vi "CFTS-Connections Dialog.vi"(2 "Parent VI":refnum<vi>) -> ()   [LabVIEW 2020]
doc: "Use this template to create a dialog box with event handling."
uses:
  epl-vi-lib/Utility VIs/Controls/KBackground Gradient/KBackground Gradient.xctl
  epl-vi-lib/Utility VIs/Controls/KTable/KTable.xctl
  CFTS-Options.ctl
  epl-vi-lib/Connection VIs/Typedefs/CM-Endpoint.ctl
  76337d95-708c-4186-8447-1f4ad4f75f43.vi
  epl-vi-lib/Utility VIs/File IO VIs/Read Write Anything/Read Anything.vi
panel:
  in  "TermConfig":bool
  in  "AO":u16(xcontrol)
  in  "AI":u16(xcontrol)
  in  "background":dbl(xcontrol)
  in  "Cancel":bool
  in  "OK":bool
  # "Connections"
  # "Outputs"
  # "Inputs"
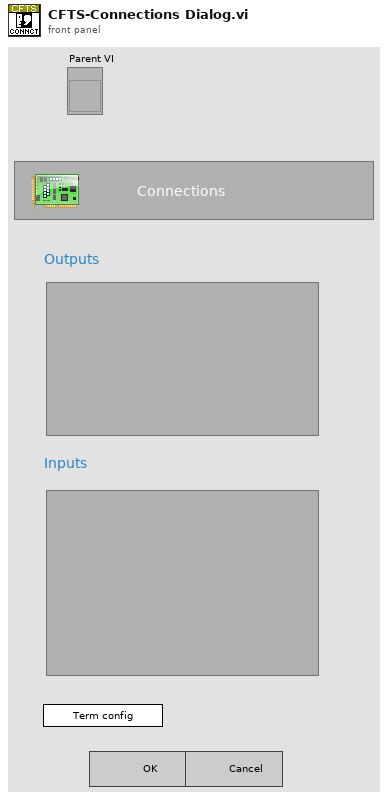
[diagram p1: front panel]
types:
  T1 = typedef "CFTS-Options.ctl" = cluster{"Rig ID":string, "Acoustic System IDs":cluster{"Right":string, "Left":string}, "Extension":string, "Advanced users":string[], "All advanced":bool, "Run vitals":bool, "hash":string, "Allow nonEPL":bool, "NonEPL":string[], "Data root":path}
  T2 = typedef "CM-Endpoint.ctl" = cluster{"Name":string, "Device":string}
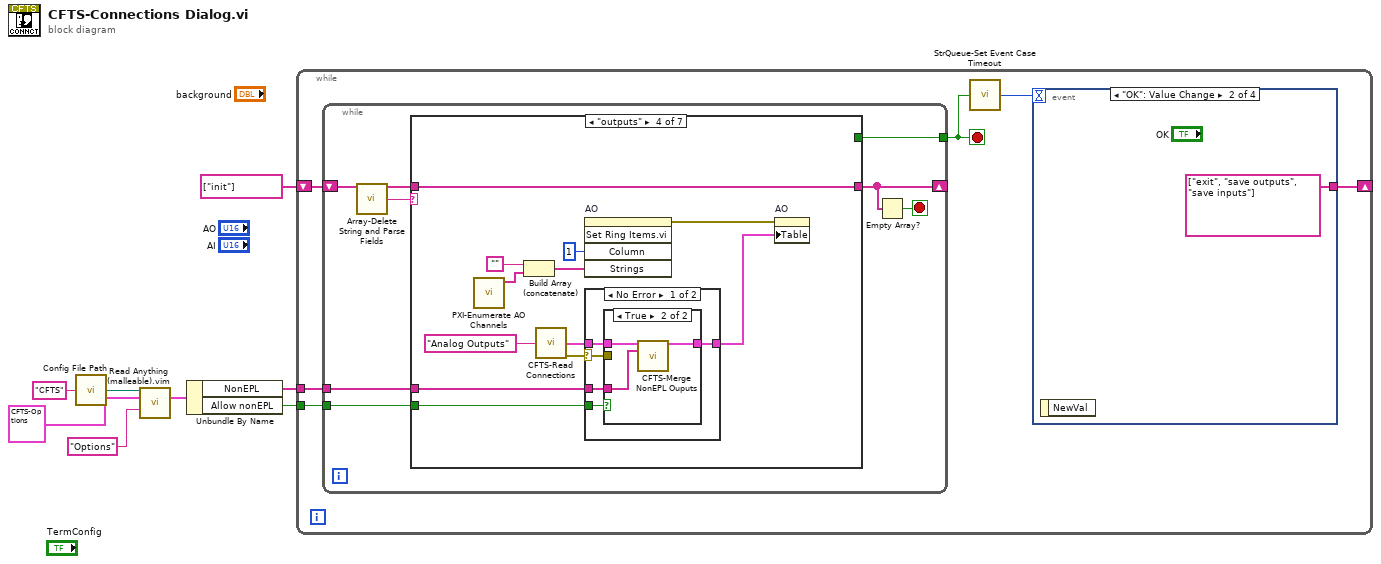
[diagram p0: block diagram]
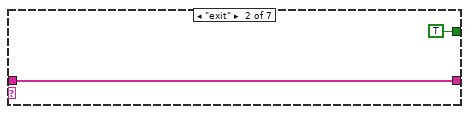
[diagram p3: hidden frame]
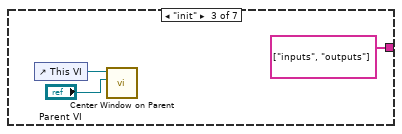
[diagram p4: hidden frame]
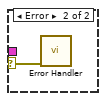
[diagram p6: hidden frame]
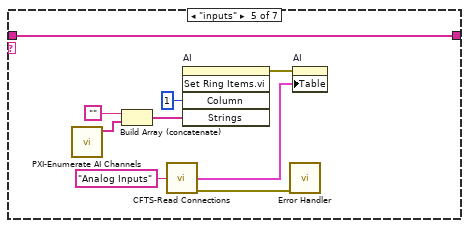
[diagram p7: hidden frame]
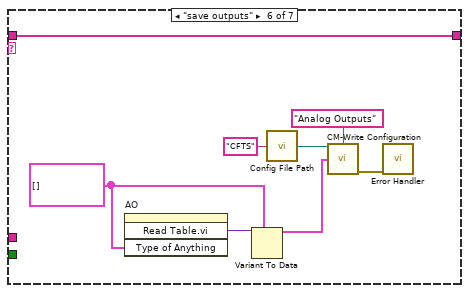
[diagram p8: hidden frame]
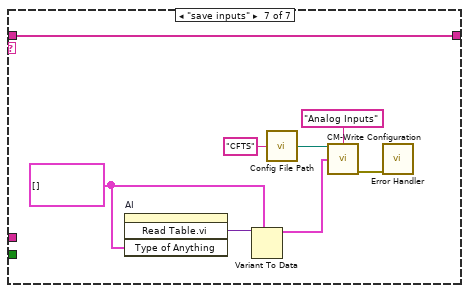
[diagram p9: hidden frame]
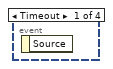
[diagram p10: hidden frame]
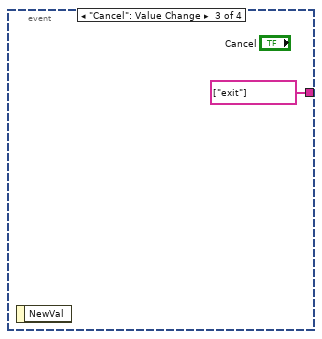
[diagram p11: hidden frame]
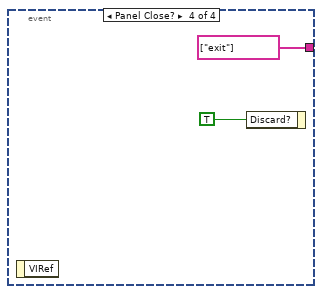
[diagram p12: hidden frame]
diagram:
  n1 = call "Config File Path.vi"("AppName"="CFTS") -> ("Default config file name"=w6:path)
  n2 = call "Read Anything (malleable).vim"("Config file path"=w6, "Options in"=T1 {"Rig ID"="", "Acoustic System IDs"={"Right"="", "Left"=""}, "Extension"="", "Advanced users"=[], "All advanced"=FALSE, "Run vitals"=FALSE, "hash"="", "Allow nonEPL"=FALSE, "NonEPL"=[], "Data root"=path ""} ("Options"), "Section"="Options") -> ("Options out"=w3:T1)  [unwired: 9 in, 3 out]
  n3 = Unbundle By Name(w3) -> ("NonEPL"=w2:string[], "Allow nonEPL"=w1:bool)
  n4 = while {
    shift-right: [w11] -> _
    shift-left: string[] ["init"] -> [w12]
    tunnel: w2 -> [w10]
    tunnel: w1 -> [w9]
    stop <- w14 stop-if-true
    n5 = while {
      shift-right: [w22] -> _
      shift-left: w12 -> [w19]
      tunnel: [w20] -> w14
      tunnel: w10 -> [w16]
      tunnel: w9 -> [w15]
      stop <- w21 stop-if-true
      n6 = call "Array-Delete String and Parse Fields.vi"("Array in"=w19) -> ("Array out"=w18:string[], "Field 1"=w17:string)  [unwired: 10 in, 3 out]
      n7 = case shown="\"outputs\"" w17 {
        tunnel: w18 -> [w23 w25 _ w40 w59 w67 w75]
        tunnel: [w23 w25 string[] ["inputs", "outputs"] ("Array out") w40 w59 w67 w75] -> w22
        tunnel: [_ TRUE _ _ _ _ _] -> w20
        tunnel: w16 -> [_ _ _ w29 _ _ _]
        tunnel: w15 -> [_ _ _ w32 _ _ _]
        frame "", Default {
        }
        frame "exit" {
        }
        frame "init" {
          n8 = control-ref of="This VI"() -> (w27:refnum<vi>)
          n9 = call "Center Window on Parent.vi"("Parent VI"="Parent VI", "VI in"=w27) -> ()  [unwired: 8 in, 2 out]
        }
        frame "outputs" {
          n10 = call "PXI-Enumerate AO Channels.vi"() -> ("AO.PhysicalChans"=w37:tag[])  [unwired: 10 in, 1 out]
          n11 = Build Array (concatenate)("", w37) -> (w35:string[])
          n12 = call "CFTS-Read Connections.vi"("Which"="Analog Outputs") -> ("endpoints"=w31:T2[], "error out"=w33:errorcluster)  [unwired: 13 in]
          n13 = invoke on="AO" class="KTable (strict)" method="Set Ring Items.vi"("Column"=1, "Strings"=w35) -> (error out=w39:errorcluster)  [unwired: 3 in, 4 out]
          n14 = case shown="No Error" w33 {
            selector: w33 -> [w45 w50]
            tunnel: w32 -> [w44 _]
            tunnel: w31 -> [w43 _]
            tunnel: [w42 _] -> w30
            tunnel: w29 -> [w41 _]
            frame No Error {
              n15 = case shown="True" w44 {
                tunnel: w45 -> [_ _]
                tunnel: w43 -> [w46 w47]
                tunnel: [w46 w48] -> w42
                tunnel: w41 -> [_ w49]
                frame False {
                }
                frame True {
                  n16 = call "CFTS-Merge NonEPL Ouputs.vi"("endpoints in"=w47, "NonEPL"=w49) -> ("endpoints out"=w48:T2[])  [unwired: 13 in]
                }
              }
            }
            frame Error {
              n17 = call "Error Handler.vi"("error in (no error)"=w50) -> ()  [unwired: 12 in, 3 out]
            }
          }
          n18 = property on="AO" class="KTable (strict)"(error in=w39, "Table"=w30) -> ()  [unwired: 1 in, 2 out]
        }
        frame "inputs" {
          n19 = call "PXI-Enumerate AI Channels.vi"() -> ("AI.PhysicalChans"=w56:tag[])  [unwired: 11 in]
          n20 = Build Array (concatenate)("", w56) -> (w54:string[])
          n21 = call "CFTS-Read Connections.vi"("Which"="Analog Inputs") -> ("endpoints"=w52:T2[], "error out"=w53:errorcluster)  [unwired: 13 in]
          n22 = invoke on="AI" class="KTable (strict)" method="Set Ring Items.vi"("Column"=1, "Strings"=w54) -> (error out=w58:errorcluster)  [unwired: 3 in, 4 out]
          n23 = call "Error Handler.vi"("error in (no error)"=w53) -> ()  [unwired: 12 in, 3 out]
          n24 = property on="AI" class="KTable (strict)"(error in=w58, "Table"=w52) -> ()  [unwired: 1 in, 2 out]
        }
        frame "save outputs" {
          w64 = T2[] [] ("Array")
          n25 = invoke on="AO" class="KTable (strict)" method="Read Table.vi"("Type of Anything"=w64) -> ("Read Table.vi"=w65:variant)  [unwired: 3 in, 3 out]
          n26 = Variant To Data(type=w64, Variant=w65) -> (data=w62:T2[])  [unwired: 1 in, 1 out]
          n27 = call "Config File Path.vi"("AppName"="CFTS") -> ("Default config file name"=w63:path)
          n28 = call "CM-Write Configuration.vi"("Connection File Path"=w63, "Section"="Analog Outputs", "Endpoints"=w62) -> ("error out"=w60:errorcluster)  [unwired: 11 in, 1 out]
          n29 = call "Error Handler.vi"("error in (no error)"=w60) -> ()  [unwired: 12 in, 3 out]
        }
        frame "save inputs" {
          w72 = T2[] [] ("Array")
          n30 = invoke on="AI" class="KTable (strict)" method="Read Table.vi"("Type of Anything"=w72) -> ("Read Table.vi"=w73:variant)  [unwired: 3 in, 3 out]
          n31 = Variant To Data(type=w72, Variant=w73) -> (data=w70:T2[])  [unwired: 1 in, 1 out]
          n32 = call "Config File Path.vi"("AppName"="CFTS") -> ("Default config file name"=w71:path)
          n33 = call "CM-Write Configuration.vi"("Connection File Path"=w71, "Section"="Analog Inputs", "Endpoints"=w70) -> ("error out"=w68:errorcluster)  [unwired: 11 in, 1 out]
          n34 = call "Error Handler.vi"("error in (no error)"=w68) -> ()  [unwired: 12 in, 3 out]
        }
      }
      n35 = Empty Array?(array=w22) -> (empty?=w21:bool)
    }
    n36 = call "StrQueue-Set Event Case Timeout.vi"("Quit"=w14) -> ("timeout"=w13:i32)  [unwired: 14 in]
    n37 = event shown="[1] \"OK\": Value Change" {
      selector: _ -> [_ _ _ _]
      dyn-events: _ -> [_ _ _ _]
      timeout: w13 -> [_ _ _ _]
      tunnel: [_ string[] ["exit", "save outputs", "save inputs"] string[] ["exit"] string[] ["exit"]] -> w11
      event Timeout {
        n38 = event-data() -> ()  [unwired: 1 in, 1 out]
      }
      event "OK": Value Change {
        n39 = event-data() -> ()  [unwired: 1 in, 1 out]
      }
      event "Cancel": Value Change {
        n40 = event-data() -> ()  [unwired: 1 in, 1 out]
      }
      event Panel Close? {
        n41 = event-data() -> ()  [unwired: 1 in, 1 out]
        n42 = event-data("Discard?"=TRUE) -> ()  [unwired: 1 in, 1 out]
      }
    }
  }
